vi "temp_val.vi"() -> (3 "return value":dbl)   [LabVIEW 2024]
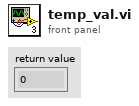
[diagram p1: front panel]
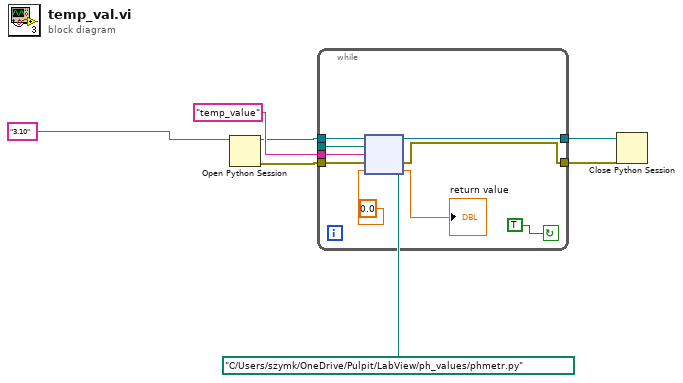
[diagram p0: block diagram]
diagram:
  n1 = Open Python Session(python version="3.10" ("Python version")) -> (session out=w2:refnum<k35>, error out=w1:errorcluster)  [unwired: 2 in]
  n2 = while {
    tunnel: w1 -> [w16]
    tunnel: w2 -> [w15]
    tunnel: "temp_value" -> [w14]
    tunnel: path "C:/Users/szymk/OneDrive/Pulpit/LabView/ph_values/phmetr.py" ("module path") -> [w13]
    tunnel: [w10] -> w6
    tunnel: [w9] -> w7
    stop <- TRUE continue-if-true
    n3 = node(w15, w13, w14, w16, 0.0) -> (w10:refnum<k35>, w9:errorcluster, →"return value":dbl)  [unwired: 2 out]
  }
  n4 = Close Python Session(session in=w6, error in=w7) -> ()  [unwired: 1 out]
